vi "Status.vi"(8 "error in (no error)":errorcluster, 9 "totalscans":u32 caption="Total Scans", 10 "scan#":u32 caption="Scan Number", 11 "Double Scanner.lvclass in":refnum<class "Double Scanner.lvclass">) -> (0 "error out":errorcluster, 2 "scanprogress":string caption="Scan Progress", 3 "Double Scanner.lvclass out":refnum<class "Double Scanner.lvclass">)   [LabVIEW 2012, in "Double Scanner.lvclass"]
doc: "(Dynamic) Return a text status message reflecting the current state of this Scanner."
uses:
  Double Scanner.lvclass
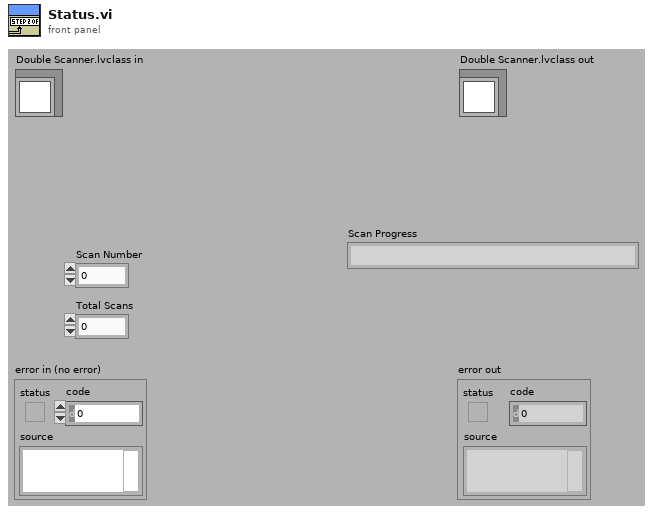
[diagram p1: front panel]
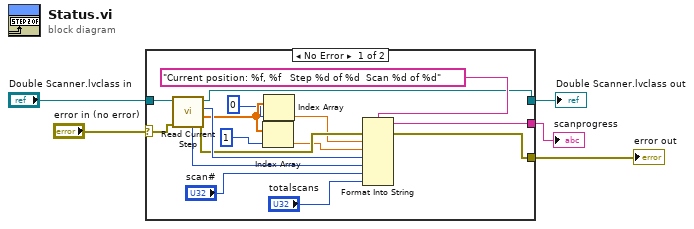
[diagram p0: block diagram]
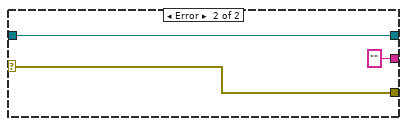
[diagram p2: hidden frame]
diagram:
  n1 = case shown="No Error" "error in (no error)" {
    selector: "error in (no error)" -> [w16 w24]
    tunnel: "Double Scanner.lvclass in" -> [w21 w23]
    tunnel: [w15 w24] -> w3
    tunnel: [w12 w23] -> w2
    tunnel: [w14 ""] -> w1
    frame No Error {
      n2 = call-dynamic "Read Current Step.vi"("error in (no error)"=w16, "Double Scanner in"=w21) -> ("error out"=w11:errorcluster, "Current Position Array"=w10:dbl[], "Current step"=w19:u32, "Double Scanner out"=w12:refnum<class "Double Scanner.lvclass">, "Total steps"=w13:i32)  [unwired: 5 in]
      n3 = Index Array(array=w10, index=1) -> (element=w6:dbl)
      n4 = Index Array(array=w10, index=0) -> (element=w7:dbl)
      n5 = Format Into String(format string="Current position: %f, %f   Step %d of %d  Scan %d of %d", error in=w11, w7, w6, w19, w13, "scan#", "totalscans") -> (resulting string=w14:string, error out=w15:errorcluster)  [unwired: 1 in]
    }
    frame Error {
    }
  }
  "error out" <- w3
  "Double Scanner.lvclass out" <- w2
  "scanprogress" <- w1
